vi "Autonomous Independent.vi"   [LabVIEW 2020]
doc: "This VI is called when autonomous begins, and will automatically be terminated when autonomous ends. You can carry out timed or sensor driven robot movement independently without needing to return to the caller."
uses:
  <vilib>/Rock Robotics/WPI/Utilities/WPI_GetSetVariantRefNum.vi
  <vilib>/Rock Robotics/Network Tables/NT Read String.vi
  <vilib>/Rock Robotics/Network Tables/NT Write Numeric Array.vi
panel:
  # "Be sure to right-click and choose Data Operations>>Make Current Value default if you want to save the array values with the VI"
types:
  T1 = typedef "WPI_JoystickDevRef.ctl" = cluster{"Device":T2}
  T2 = typedef "WPI_JoystickDeviceEnum.ctl" = enum16{"USB 0", "USB 1", "USB 2", "USB 3", "USB 4", "USB 5"}
  T3 = typedef "WPI_RobotDriveDevRef.ctl" = cluster{"DevStatus":errorcluster, "Motors[]":T4[], "Square Inputs":bool, "Max Output":dbl}
  T4 = typedef "WPI_MotorControlDeviceRef.ctl" = cluster{"DeviceStatus":errorcluster, "Type":T5, "PWM":cluster{"PWM Channel":T6, "DeadBand":T7}, "CAN":cluster{"Device Number":u8, "SetOutput VI Ref":variant, "GetOutput VI Ref":variant, "Enable VI Ref":variant, "Disable VI Ref":variant, "Data":variant}, "Invert":bool, "DIO PWM":cluster{"PWM \"Enable\" Channel":T6, "DIOChannel":T8, "PWM Rate":dbl}}
  T5 = typedef "WPI_MotorControlType.ctl" = enum16{"PWM", "CAN", "DIO PWM"}
  T6 = typedef "FPGA_DIOPWMChannel.ctl" = enum8{"PWM 0", "PWM 1", "PWM 2", "PWM 3", "PWM 4", "PWM 5", "PWM 6", "PWM 7", "PWM 8", "PWM 9", "PWM MXP 0", "PWM MXP 1", "PWM MXP 2", "PWM MXP 3", "PWM MXP 4", "PWM MXP 5", "PWM MXP 6", "PWM MXP 7", "PWM MXP 8", "PWM MXP 9", "Invalid"}
  T7 = typedef "WPI_PWMDeadband.ctl" = cluster{"Name":string, "maxPositivePwm":i32, "minPositivePwm":i32, "centerPwm":i32, "maxNegativePwm":i32, "minNegativePwm":i32, "angularRange":u16}
  T8 = typedef "FPGA_DIOChannel.ctl" = enum8{"DIO 0", "DIO 1", "DIO 2", "DIO 3", "DIO 4", "DIO 5", "DIO 6", "DIO 7", "DIO 8", "DIO 9", "DIO MXP 0", "DIO MXP 1", "DIO MXP 2", "DIO MXP 3", "DIO MXP 4", "DIO MXP 5", "DIO MXP 6", "DIO MXP 7", "DIO MXP 8", "DIO MXP 9", "DIO MXP 10", "DIO MXP 11", "DIO MXP 12", "DIO MXP 13", "DIO MXP 14", "DIO MXP 15", "SPI Port CS1", "SPI Port CS2", "SPI Port CS3", "SPI Port MISO", "SPI Port MOSI", "Invalid"}
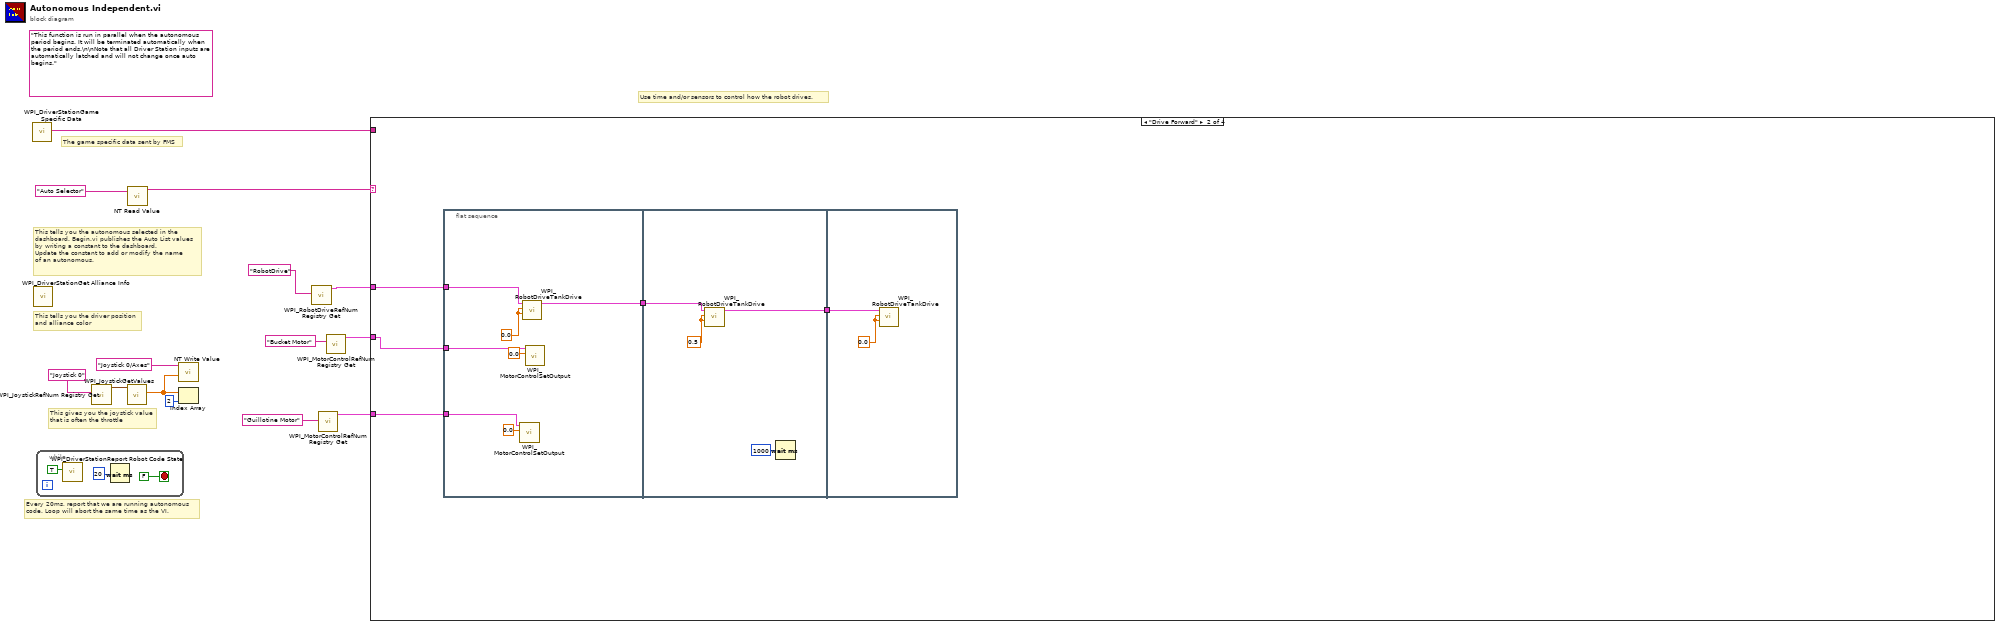
[diagram p0: block diagram]
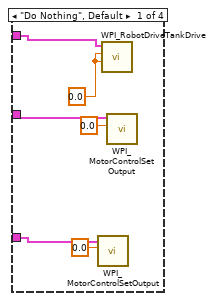
[diagram p2: hidden frame]
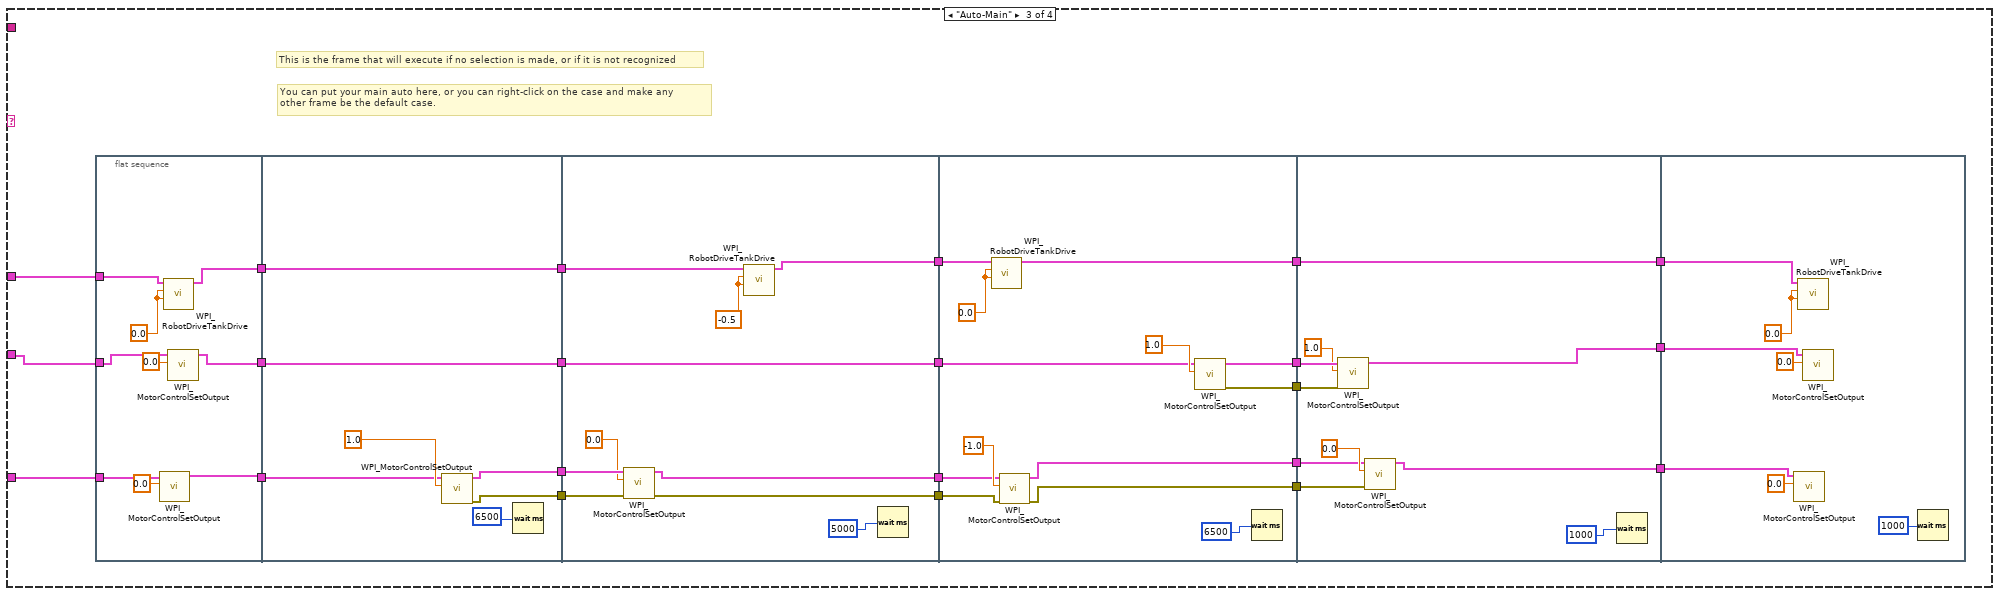
[diagram p3: hidden frame]
diagram:
  (unwired) "This function is run in parallel when the autonomous period begins. It will be terminated automatically when the period ends.\n\nNote that all Driver Station inputs are automatically latched and will not change once auto begins."
  # "The game specific data sent by FMS"
  # "This tells you the autonomous selected in the \ndashboard. Begin.vi publishes the Auto List values\nby writing a constant to the dashboard.\nUpdate the constant to add or modify the name\nof an autonomous."
  # "Every 20ms, report that we are running autonomous\ncode. Loop will abort the same time as the VI."
  # "This gives you the joystick value\nthat is often the throttle"
  # "Use time and/or sensors to control how the robot drives."
  # "This tells you the driver position\nand alliance color"
  n1 = call <vilib>:"WPI_DriverStationGame Specific Data.vi"() -> ("Game Specific Data"=w7:string)  [unwired: 11 in]
  n2 = call <vilib>:"WPI_DriverStationGet Alliance Info.vi"() -> ()  [unwired: 12 out]
  n3 = while {
    stop <- FALSE stop-if-true
    n4 = call <vilib>:"WPI_DriverStationReport Robot Code State.vi"("Autonomous"=TRUE) -> ()  [unwired: 10 in, 1 out]
    n5 = Wait (ms)(milliseconds to wait=u32 20) -> ()  [unwired: 1 out]
  }
  n6 = call <vilib>:"WPI_JoystickRefNum Registry Get.vi"("refnum name"="Joystick 0") -> ("JoystickDevRef"=w13:T1)  [unwired: 1 in, 9 out]
  n7 = call <vilib>:"WPI_JoystickGetValues.vi"("JoystickDevRef"=w13) -> ("Axes"=w9:dbl[])  [unwired: 6 in, 4 out]
  n8 = call-poly <vilib>:"NT Read Value.vi"("Name"="Auto Selector") -> ("String"=w10:string)  [unwired: 9 in, 1 out]
  n9 = call-poly <vilib>:"NT Write Value.vi"("Numeric Array"=w9, "Name"="Joystick 0/Axes") -> ()  [unwired: 9 in, 1 out]
  n10 = Index Array(array=w9, index=2) -> ()  [unwired: 1 out]
  n11 = call <vilib>:"WPI_RobotDriveRefNum Registry Get.vi"("refnum name"="RobotDrive") -> ("RobotDriveDevRef"=w6:T3)  [unwired: 1 in, 9 out]
  n12 = call <vilib>:"WPI_MotorControlRefNum Registry Get.vi"("refnum name"="Guillotine Motor") -> ("MotorControlDevRef"=w4:T4)  [unwired: 9 in, 1 out]
  n13 = call <vilib>:"WPI_MotorControlRefNum Registry Get.vi"("refnum name"="Bucket Motor") -> ("MotorControlDevRef"=w1:T4)  [unwired: 9 in, 1 out]
  n14 = case shown="\"Drive Forward\"" w10 {
    tunnel: w7 -> [_ _ _ _]
    tunnel: w6 -> [w20 w28 w54 _]
    tunnel: w4 -> [w18 w26 w53 _]
    tunnel: w1 -> [w19 w27 w52 _]
    frame "Do Nothing", Default {
      w23 = 0.0
      n15 = call <vilib>:"WPI_MotorControlSetOutput.vi"("Output"=0.0, "MotorControlDevRef"=w18) -> ()  [unwired: 7 in, 3 out]
      n16 = call <vilib>:"WPI_RobotDriveTankDrive.vi"("Right axis value"=w23, "Left axis value"=w23, "RobotDriveDevRef"=w20) -> ()  [unwired: 6 in, 3 out]
      n17 = call <vilib>:"WPI_MotorControlSetOutput.vi"("Output"=0.0, "MotorControlDevRef"=w19) -> ()  [unwired: 7 in, 3 out]
    }
    frame "Drive Forward" {
      n18 = flat-sequence {
        tunnel: w28 -> [w32]
        tunnel: w27 -> [w31]
        tunnel: w26 -> [w30]
        tunnel: [w29] -> w25
        tunnel: w25 -> [w38]
        tunnel: [w36] -> w24
        tunnel: w24 -> [w40]
        frame #0 {
          w35 = 0.0
          n19 = call <vilib>:"WPI_MotorControlSetOutput.vi"("Output"=0.0, "MotorControlDevRef"=w30) -> ()  [unwired: 7 in, 3 out]
          n20 = call <vilib>:"WPI_RobotDriveTankDrive.vi"("Right axis value"=w35, "Left axis value"=w35, "RobotDriveDevRef"=w32) -> ("RobotDriveDevRef"=w29:T3)  [unwired: 6 in, 2 out]
          n21 = call <vilib>:"WPI_MotorControlSetOutput.vi"("Output"=0.0, "MotorControlDevRef"=w31) -> ()  [unwired: 7 in, 3 out]
        }
        frame #1 {
          w39 = 0.5
          n22 = call <vilib>:"WPI_RobotDriveTankDrive.vi"("Right axis value"=w39, "Left axis value"=w39, "RobotDriveDevRef"=w38) -> ("RobotDriveDevRef"=w36:T3)  [unwired: 6 in, 2 out]
          n23 = Wait (ms)(milliseconds to wait=u32 1000) -> ()  [unwired: 1 out]
        }
        frame #2 {
          w41 = 0.0
          n24 = call <vilib>:"WPI_RobotDriveTankDrive.vi"("Right axis value"=w41, "Left axis value"=w41, "RobotDriveDevRef"=w40) -> ()  [unwired: 6 in, 3 out]
        }
      }
    }
    frame "Auto-Main" {
      # "You can put your main auto here, or you can right-click on the case and make any\nother frame be the default case."
      # "This is the frame that will execute if no selection is made, or if it is not recognized"
      n25 = flat-sequence {
        tunnel: w52 -> [w70]
        tunnel: w53 -> [w68]
        tunnel: w54 -> [w71]
        tunnel: [w67] -> w51
        tunnel: [w69] -> w48
        tunnel: [w64] -> w46
        tunnel: [w77] -> w63
        tunnel: [w76] -> w62
        tunnel: w51 -> [w75]
        tunnel: [w74] -> w49
        tunnel: w48 -> [w74]
        tunnel: [w73] -> w47
        tunnel: w46 -> [w73]
        tunnel: w63 -> [w88]
        tunnel: w62 -> [w87]
        tunnel: [w85] -> w61
        tunnel: [w84] -> w60
        tunnel: [w82] -> w57
        tunnel: [w81] -> w50
        tunnel: w49 -> [w81]
        tunnel: w47 -> [w80]
        tunnel: w61 -> [w100]
        tunnel: w60 -> [w99]
        tunnel: [w98] -> w59
        tunnel: [w97] -> w58
        tunnel: w57 -> [w95]
        tunnel: [w93] -> w56
        tunnel: [w92] -> w55
        tunnel: w50 -> [w91]
        tunnel: [w90] -> w45
        tunnel: w59 -> [w110]
        tunnel: w58 -> [w109]
        tunnel: w56 -> [w108]
        tunnel: w55 -> [w107]
        tunnel: w45 -> [w105]
        tunnel: [w105] -> w44
        tunnel: [w104] -> w43
        tunnel: [w103] -> w42
        tunnel: w44 -> [w115]
        tunnel: w43 -> [w114]
        tunnel: w42 -> [w113]
        frame #0 {
          w72 = 0.0
          n26 = call <vilib>:"WPI_MotorControlSetOutput.vi"("Output"=0.0, "MotorControlDevRef"=w68) -> ("MotorControlDevRef"=w67:T4)  [unwired: 7 in, 2 out]
          n27 = call <vilib>:"WPI_RobotDriveTankDrive.vi"("Right axis value"=w72, "Left axis value"=w72, "RobotDriveDevRef"=w71) -> ("RobotDriveDevRef"=w64:T3)  [unwired: 6 in, 2 out]
          n28 = call <vilib>:"WPI_MotorControlSetOutput.vi"("Output"=0.0, "MotorControlDevRef"=w70) -> ("MotorControlDevRef"=w69:T4)  [unwired: 7 in, 2 out]
        }
        frame #1 {
          n29 = call <vilib>:"WPI_MotorControlSetOutput.vi"("Output"=1.0, "MotorControlDevRef"=w75) -> ("error out"=w76:errorcluster, "MotorControlDevRef"=w77:T4)  [unwired: 7 in, 1 out]
          n30 = Wait (ms)(milliseconds to wait=u32 6500) -> ()  [unwired: 1 out]
        }
        frame #2 {
          w83 = -0.5
          n31 = call <vilib>:"WPI_MotorControlSetOutput.vi"("error in (no error)"=w87, "Output"=0.0, "MotorControlDevRef"=w88) -> ("error out"=w84:errorcluster, "MotorControlDevRef"=w85:T4)  [unwired: 6 in, 1 out]
          n32 = call <vilib>:"WPI_RobotDriveTankDrive.vi"("Right axis value"=w83, "Left axis value"=w83, "RobotDriveDevRef"=w80) -> ("RobotDriveDevRef"=w82:T3)  [unwired: 6 in, 2 out]
          n33 = Wait (ms)(milliseconds to wait=u32 5000) -> ()  [unwired: 1 out]
        }
        frame #3 {
          w96 = 0.0
          n34 = call <vilib>:"WPI_RobotDriveTankDrive.vi"("Right axis value"=w96, "Left axis value"=w96, "RobotDriveDevRef"=w95) -> ("RobotDriveDevRef"=w90:T3)  [unwired: 6 in, 2 out]
          n35 = call <vilib>:"WPI_MotorControlSetOutput.vi"("error in (no error)"=w99, "Output"=-1.0, "MotorControlDevRef"=w100) -> ("error out"=w97:errorcluster, "MotorControlDevRef"=w98:T4)  [unwired: 6 in, 1 out]
          n36 = call <vilib>:"WPI_MotorControlSetOutput.vi"("Output"=1.0, "MotorControlDevRef"=w91) -> ("error out"=w92:errorcluster, "MotorControlDevRef"=w93:T4)  [unwired: 7 in, 1 out]
          n37 = Wait (ms)(milliseconds to wait=u32 6500) -> ()  [unwired: 1 out]
        }
        frame #4 {
          n38 = call <vilib>:"WPI_MotorControlSetOutput.vi"("error in (no error)"=w107, "Output"=1.0, "MotorControlDevRef"=w108) -> ("MotorControlDevRef"=w104:T4)  [unwired: 6 in, 2 out]
          n39 = call <vilib>:"WPI_MotorControlSetOutput.vi"("error in (no error)"=w109, "Output"=0.0, "MotorControlDevRef"=w110) -> ("MotorControlDevRef"=w103:T4)  [unwired: 6 in, 2 out]
          n40 = Wait (ms)(milliseconds to wait=u32 1000) -> ()  [unwired: 1 out]
        }
        frame #5 {
          w118 = 0.0
          n41 = call <vilib>:"WPI_MotorControlSetOutput.vi"("Output"=0.0, "MotorControlDevRef"=w113) -> ()  [unwired: 7 in, 3 out]
          n42 = call <vilib>:"WPI_RobotDriveTankDrive.vi"("Right axis value"=w118, "Left axis value"=w118, "RobotDriveDevRef"=w115) -> ()  [unwired: 6 in, 3 out]
          n43 = call <vilib>:"WPI_MotorControlSetOutput.vi"("Output"=0.0, "MotorControlDevRef"=w114) -> ()  [unwired: 7 in, 3 out]
          n44 = Wait (ms)(milliseconds to wait=u32 1000) -> ()  [unwired: 1 out]
        }
      }
    }
    frame "Fancy-Auto" {
    }
  }
